vi "PPR_TRAJ_ABS_POSE_EST_BEGIN.vi"(8 "error in (no error)":errorcluster, 9 "Initial Pose":T1 {"ROTATION"."SIN" format="%13.4f"; "ROTATION"."COS" format="%13.4f"; "ROTATION"."VALUE" format="%13.4f"; "TRANSLATION"."Y" format="%14.3f"; "TRANSLATION"."X" format="%14.3f"}, 10 "Initial Gyro Angle":T3 {"SIN" format="%13.4f"; "COS" format="%13.4f"; "VALUE" format="%13.4f"}) -> (0 "error out":errorcluster)   [LabVIEW 2019]
uses:
  PPR_TRAJECTORY_GLOBALS.vi
  <vilib>/Rock Robotics/WPI/ThirdParty/JAS_Junk/TrajLib/Trajectory_Library.lvlib
  <vilib>/Rock Robotics/WPI/ThirdParty/JAS_Junk/TrajLib/TypeDef/ROTATION2D.ctl
  <vilib>/Rock Robotics/WPI/ThirdParty/JAS_Junk/TrajLib/TypeDef/TRANSLATION2D.ctl
  <vilib>/Rock Robotics/WPI/ThirdParty/JAS_Junk/TrajLib/TypeDef/POSE2D.ctl
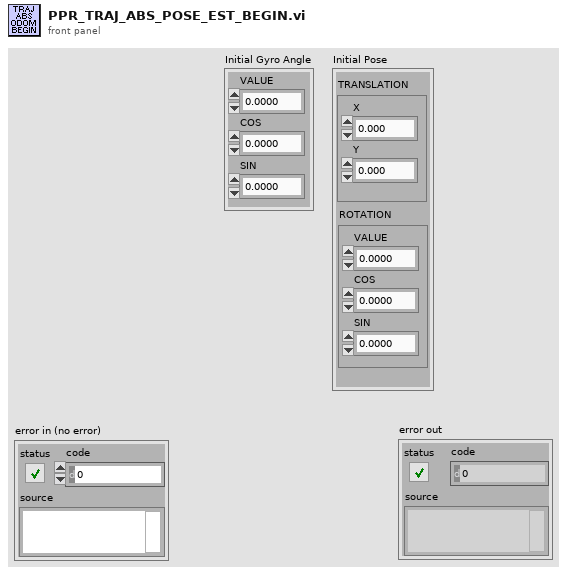
[diagram p1: front panel]
types:
  T1 = typedef "Trajectory_Library.lvlib/POSE2D.ctl" = cluster{"TRANSLATION":T2, "ROTATION":T3}
  T2 = typedef "Trajectory_Library.lvlib/TRANSLATION2D.ctl" = cluster{"X":dbl, "Y":dbl}
  T3 = typedef "Trajectory_Library.lvlib/ROTATION2D.ctl" = cluster{"VALUE":dbl, "COS":dbl, "SIN":dbl}
  T4 = typedef "Trajectory_Library.lvlib/DIFF_DRIVE_ODOM2.ctl" = cluster{"M_POSE_Meters":T1, "M_GyroOffset":T3, "M_PrevAngle":T3, "M_PrevLeftDist_M":dbl, "M_PrevRightDist_M":dbl, "M_InitLeftDist_M":dbl, "M_InitRightDist_M":dbl}
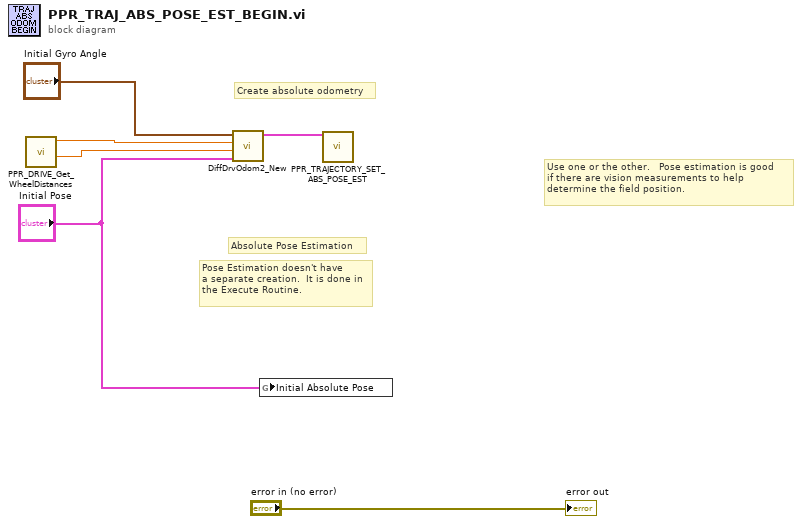
[diagram p0: block diagram]
diagram:
  # "Create absolute odometry"
  # "Absolute Pose Estimation"
  # "Pose Estimation doesn't have\na separate creation.  It is done in\nthe Execute Routine."
  # "Use one or the other.   Pose estimation is good\nif there are vision measurements to help\ndetermine the field position."
  n1 = call "PPR_DRIVE_Get_WheelDistances.vi"() -> ("Right Wheel Dist M"=w1:dbl, "Left Wheel Dist M"=w4:dbl)  [unwired: 10 in]
  n2 = call <vilib>:"DiffDrvOdom2_New.vi"("Initial Pose Meters"="Initial Pose", "Initial Right Distance M"=w1, "Initial Left Distance M"=w4, "Initial Gyro Reading"="Initial Gyro Angle") -> ("Out DIFF_DRIVE_ODOM"=w2:T4)  [unwired: 7 in]
  n3 = global write "PPR_TRAJECTORY_GLOBALS.vi" "Initial Absolute Pose"("Initial Pose") -> ()
  n4 = call "PPR_TRAJECTORY_SET_ABS_POSE_EST.vi"("Absolue Odometry"=w2) -> ()  [unwired: 11 in]
  "error out" <- "error in (no error)"
